vi "sacar_datos.vi"() -> ()   [LabVIEW 2018]
panel:
  out "Dato3 2":sgl
  out "Dato3":sgl
  out "Dato2":sgl
  out "concatenated string 3":string
  out "concatenated string 2":string
  out "Dato1":sgl
  out "concatenated string":string
  out "sensor3":string
  out "sensor2":string
  out "sensor1":string
  in  "Dato":string
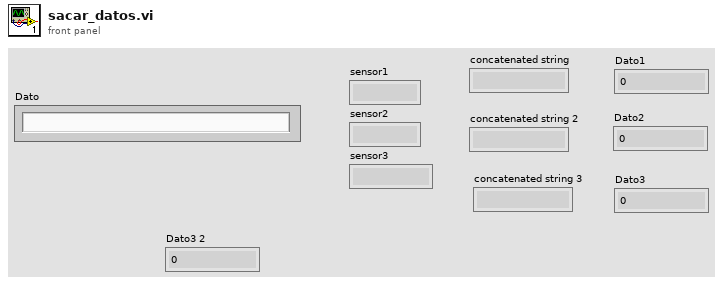
[diagram p1: front panel]
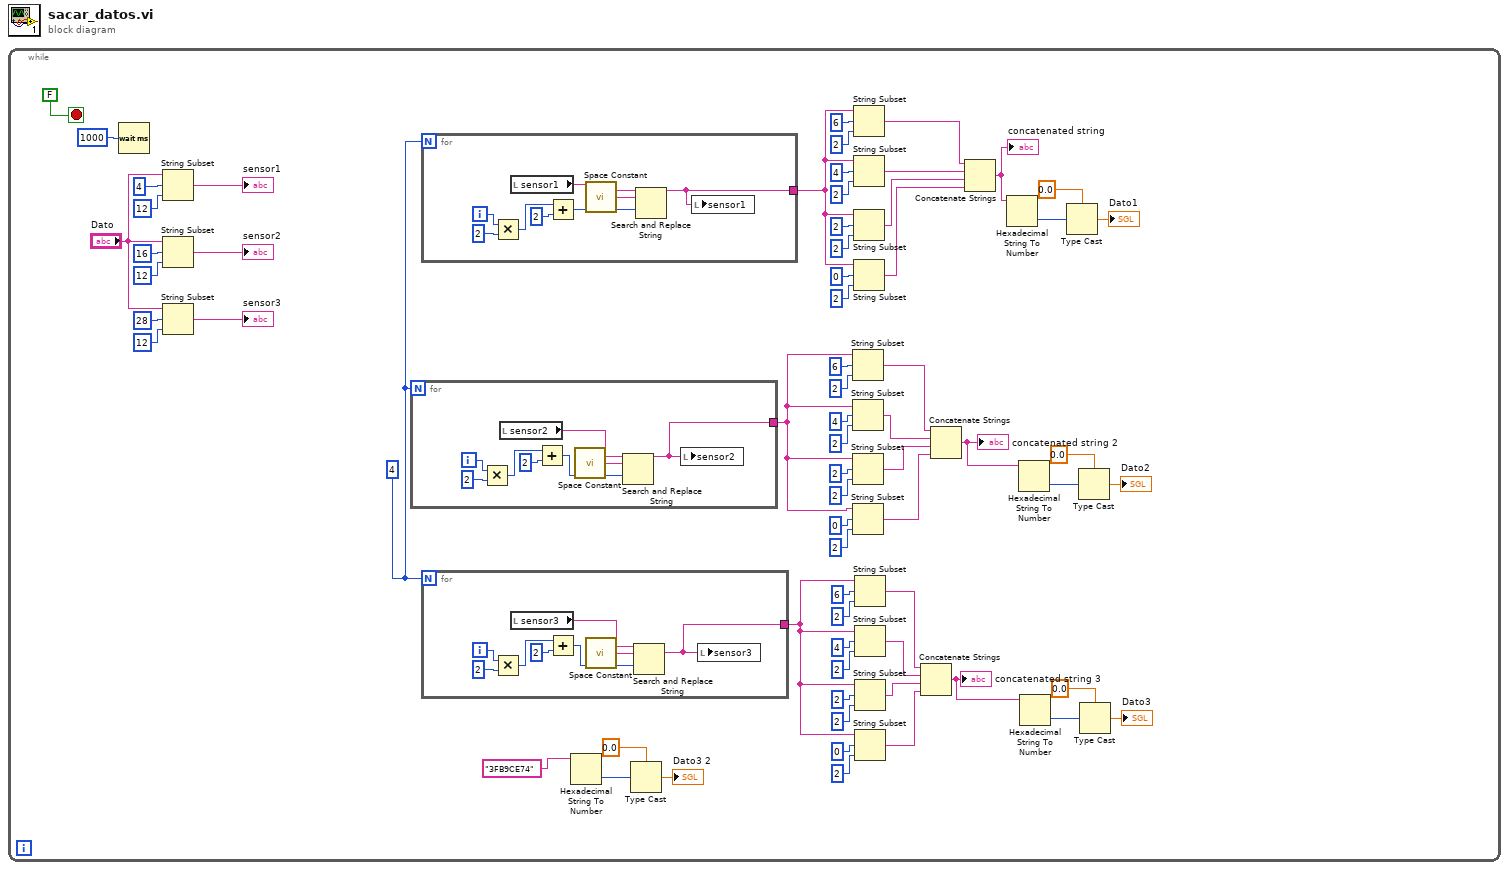
[diagram p0: block diagram]
diagram:
  n1 = while {
    stop <- FALSE stop-if-true
    w57 = 4
    n2 = Wait (ms)(milliseconds to wait=u32 1000) -> ()  [unwired: 1 out]
    n3 = String Subset(string="Dato", offset (0)=4, length (rest)=12 ("length (len. of substring)")) -> (substring=→"sensor1":string)
    n4 = String Subset(string="Dato", offset (0)=16, length (rest)=12 ("length (len. of substring)")) -> (substring=→"sensor2":string)
    n5 = String Subset(string="Dato", offset (0)=28, length (rest)=12 ("length (len. of substring)")) -> (substring=→"sensor3":string)
    n6 = for {
      N: w57 -> [_]
      tunnel: [w85] -> w30
      i -> [w91]
      n7 = Multiply(x=w91, y=2) -> (x*y=w89:i32)
      n8 = local read "sensor2"() -> (w92:string)
      n9 = Add(x=w89, y=2) -> (x+y=w87:i32)
      n10 = call <vilib>:"Space Constant.vi"() -> ("String"=w86:string)
      n11 = Search and Replace String(input string=w92, search string=w86, offset=w87) -> (result string=w85:string)  [unwired: 5 in, 3 out]
      n12 = local write "sensor2"(w85) -> ()
    }
    n13 = for {
      N: w57 -> [_]
      tunnel: [w77] -> w48
      i -> [w83]
      n14 = Multiply(x=w83, y=2) -> (x*y=w81:i32)
      n15 = local read "sensor1"() -> (w84:string)
      n16 = Add(x=w81, y=2) -> (x+y=w79:i32)
      n17 = call <vilib>:"Space Constant.vi"() -> ("String"=w78:string)
      n18 = Search and Replace String(input string=w84, search string=w78, offset=w79) -> (result string=w77:string)  [unwired: 5 in, 3 out]
      n19 = local write "sensor1"(w77) -> ()
    }
    n20 = for {
      N: w57 -> [_]
      tunnel: [w69] -> w17
      i -> [w75]
      n21 = Multiply(x=w75, y=2) -> (x*y=w73:i32)
      n22 = local read "sensor3"() -> (w76:string)
      n23 = Add(x=w73, y=2) -> (x+y=w71:i32)
      n24 = call <vilib>:"Space Constant.vi"() -> ("String"=w70:string)
      n25 = Search and Replace String(input string=w76, search string=w70, offset=w71) -> (result string=w69:string)  [unwired: 5 in, 3 out]
      n26 = local write "sensor3"(w69) -> ()
    }
    n27 = Hexadecimal String To Number(string="3FB9CE74" ("Dato")) -> (number=w2:u32)  [unwired: 2 in, 1 out]
    n28 = Type Cast(type=sgl 0.0 ("Numeric"), x=w2) -> (*(type *) &x=→"Dato3 2":sgl)
    n29 = String Subset(string=w30, offset (0)=6, length (rest)=2 ("length (rest)")) -> (substring=w29:string)
    n30 = String Subset(string=w30, offset (0)=4, length (rest)=2 ("length (rest)")) -> (substring=w28:string)
    n31 = String Subset(string=w30, offset (0)=2, length (rest)=2 ("length (rest)")) -> (substring=w27:string)
    n32 = String Subset(string=w30, offset (0)=0, length (rest)=2 ("length (rest)")) -> (substring=w26:string)
    n33 = String Subset(string=w48, offset (0)=6, length (rest)=2 ("length (rest)")) -> (substring=w45:string)
    n34 = String Subset(string=w48, offset (0)=4, length (rest)=2 ("length (rest)")) -> (substring=w44:string)
    n35 = String Subset(string=w48, offset (0)=2, length (rest)=2 ("length (rest)")) -> (substring=w47:string)
    n36 = String Subset(string=w48, offset (0)=0, length (rest)=2 ("length (rest)")) -> (substring=w46:string)
    n37 = String Subset(string=w17, offset (0)=6, length (rest)=2 ("length (rest)")) -> (substring=w16:string)
    n38 = String Subset(string=w17, offset (0)=4, length (rest)=2 ("length (rest)")) -> (substring=w15:string)
    n39 = String Subset(string=w17, offset (0)=2, length (rest)=2 ("length (rest)")) -> (substring=w14:string)
    n40 = String Subset(string=w17, offset (0)=0, length (rest)=2 ("length (rest)")) -> (substring=w13:string)
    n41 = Concatenate Strings(w16, w15, w14, w13) -> (w7:string)
    "concatenated string 3" <- w7
    n42 = Concatenate Strings(w29, w28, w27, w26) -> (w9:string)
    "concatenated string 2" <- w9
    n43 = Concatenate Strings(w45, w44, w47, w46) -> (w41:string)
    "concatenated string" <- w41
    n44 = Hexadecimal String To Number(string=w41) -> (number=w40:u32)  [unwired: 2 in, 1 out]
    n45 = Hexadecimal String To Number(string=w9) -> (number=w12:u32)  [unwired: 2 in, 1 out]
    n46 = Hexadecimal String To Number(string=w7) -> (number=w8:u32)  [unwired: 2 in, 1 out]
    n47 = Type Cast(type=sgl 0.0 ("Numeric"), x=w40) -> (*(type *) &x=→"Dato1":sgl)
    n48 = Type Cast(type=sgl 0.0 ("Numeric"), x=w12) -> (*(type *) &x=→"Dato2":sgl)
    n49 = Type Cast(type=sgl 0.0 ("Numeric"), x=w8) -> (*(type *) &x=→"Dato3":sgl)
  }
